vi "CopyPixmapToImageFlattenMaskARGB.vi"(7 "Colour (Default: Black)":T1={"Alpha"=255, "RGB"=0}, 8 "error in (no error)":errorcluster, 10 "ARGB Image Destination":refnum<data-value>, 11 "Pixmap Image Data":T2) -> (0 "error out":errorcluster, 3 "ARGB Image Destination (duplicate)":refnum<data-value>)   [LabVIEW 2020, in "g_ar_toolkit.image.lvlib"]
uses:
  g_ar_toolkit.image.lvlib
  80b1166a-8c06-443b-b271-eb6a715622f7.vi
  <vilib>/picture/picture.llb/imagedata.ctl
  ARGB Colour.ctl
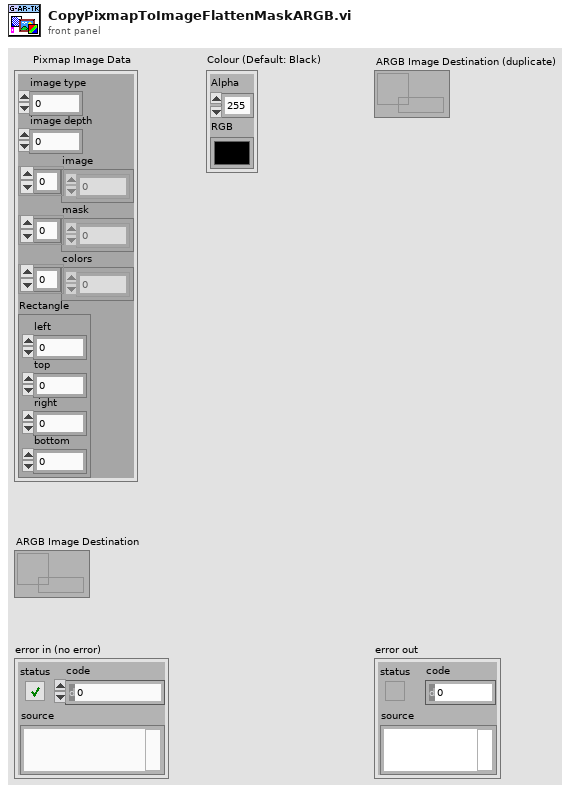
[diagram p1: front panel]
types:
  T1 = typedef "g_ar_toolkit.image.lvlib/ARGB Colour.ctl" = cluster{"Alpha":u8, "RGB":u32}
  T2 = typedef "imagedata.ctl" = cluster{"image type":i32, "image depth":i32, "image":u8[], "mask":u8[], "colors":u32[], "Rectangle":cluster{"left":i16, "top":i16, "right":i16, "bottom":i16}}
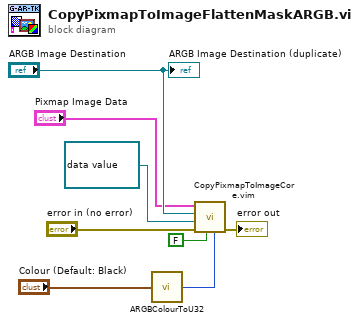
[diagram p0: block diagram]
diagram:
  n1 = call "ARGBColourToU32.vi"("ARGB Colour"="Colour (Default: Black)") -> ("U32 Colour"=w1:u32)
  n2 = call "CopyPixmapToImageCore.vim"("Background Value"=w1, "Has Mask"=FALSE, "error in (no error)"="error in (no error)", "Mask Image"=refnum<data-value> refnum ("ARGB Image Mask"), "Destination Image"="ARGB Image Destination", "image data"="Pixmap Image Data") -> ("error out"=→"error out":errorcluster)  [unwired: 5 in]
  "ARGB Image Destination (duplicate)" <- "ARGB Image Destination"
